vi "Untitled 3.vi"   [LabVIEW 2017]
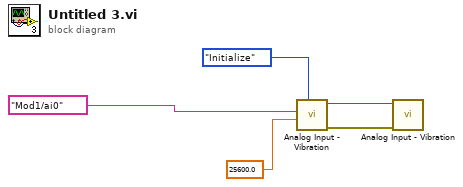
[diagram p0: block diagram]
diagram:
  n1 = call "Analog Input - Vibration.vi"("Action"=enum16{"Initialize", "Read", "Close"}."Initialize" ("Enum"), "Sample Rate"=25600.0, "Channel"=tag "Mod1/ai0") -> ("error out"=w3:errorcluster, "task out"=w4:refnum<k21>)  [unwired: 6 in, 1 out]
  n2 = call "Analog Input - Vibration.vi"("error in (no error)"=w3, "task in"=w4) -> ()  [unwired: 7 in, 3 out]
